vi "VSG25_FM.vi"(0 "Device Handle In":i32, 1 "Run as Subpanel":bool, 2 "FM Cluster In":T1={"Carrier Freq"=1.0, "Baseband Freq"=15.0, "Carrier Hz"=3, "Baseband Hz"=1, "Deviation Freq"=75.0, "Deviation Hz"=1, "Amplitude"=-10.0, "Modulation Shape"=0} {"Modulation Shape" items=["Sine Wave", "Triangle Wave", "Square Wave", "Ramp Wave"]; "Carrier Hz" items=["Hz", "kHz", "MHz", "GHz"]; "Baseband Hz" items=["Hz", "kHz", "MHz", "GHz"]; "Deviation Hz" items=["Hz", "kHz", "MHz", "GHz"]}, 3 "Error In":errorcluster) -> (5 "Device Handle Out":i32, 6 "FM Cluster Out":T1 {"Modulation Shape" items=["Sine Wave", "Triangle Wave", "Square Wave", "Ramp Wave"]; "Carrier Hz" items=["Hz", "kHz", "MHz", "GHz"]; "Baseband Hz" items=["Hz", "kHz", "MHz", "GHz"]; "Deviation Hz" items=["Hz", "kHz", "MHz", "GHz"]}, 7 "Error Out":errorcluster)   [LabVIEW 2014]
uses:
  Frequency Hertz.ctl
  Shape Control.ctl
  FM Cluster.ctl
  sg_lib/VSG25A.lvlib
panel:
  in  "Stop":bool
  out "Device Selected":bool
  in  "Modulation Shape":T3 items=["Sine Wave", "Triangle Wave", "Square Wave", "Ramp Wave"]
  in  "Deviation Hz":T2 items=["Hz", "kHz", "MHz", "GHz"]
  in  "FM Deviation":dbl
  in  "Baseband Hz":T2 items=["Hz", "kHz", "MHz", "GHz"]
  in  "Baseband Frequency":dbl
  in  "RF On":bool
  in  "Carrier Hz":T2 items=["Hz", "kHz", "MHz", "GHz"]
  in  "Amplitude (dBm)":dbl
  in  "Carrier Frequency":dbl
  # "Frequency Modulation"
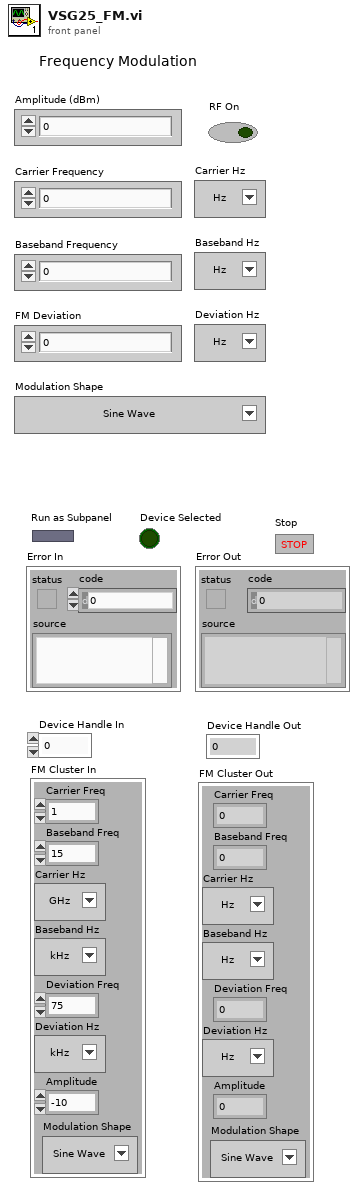
[diagram p1: front panel]
types:
  T1 = typedef "FM Cluster.ctl" = cluster{"Carrier Freq":dbl, "Baseband Freq":dbl, "Carrier Hz":T2, "Baseband Hz":T2, "Deviation Freq":dbl, "Deviation Hz":T2, "Amplitude":dbl, "Modulation Shape":T3}
  T2 = typedef "Frequency Hertz.ctl" = u16
  T3 = typedef "Shape Control.ctl" = u16
  T4 = enum16{"Init", "Proc Events", "Write VSG25", "Exit"}
  T5 = enum32{"Bad", "Idle", "Run top level", "Running"}
  T6 = enum16{"Check Amplitude ", "Check Carrier", "Check Baseband", "Check Deviation", "Stop RF", "Set Freq and Amp", "Set FM", "Finish"}
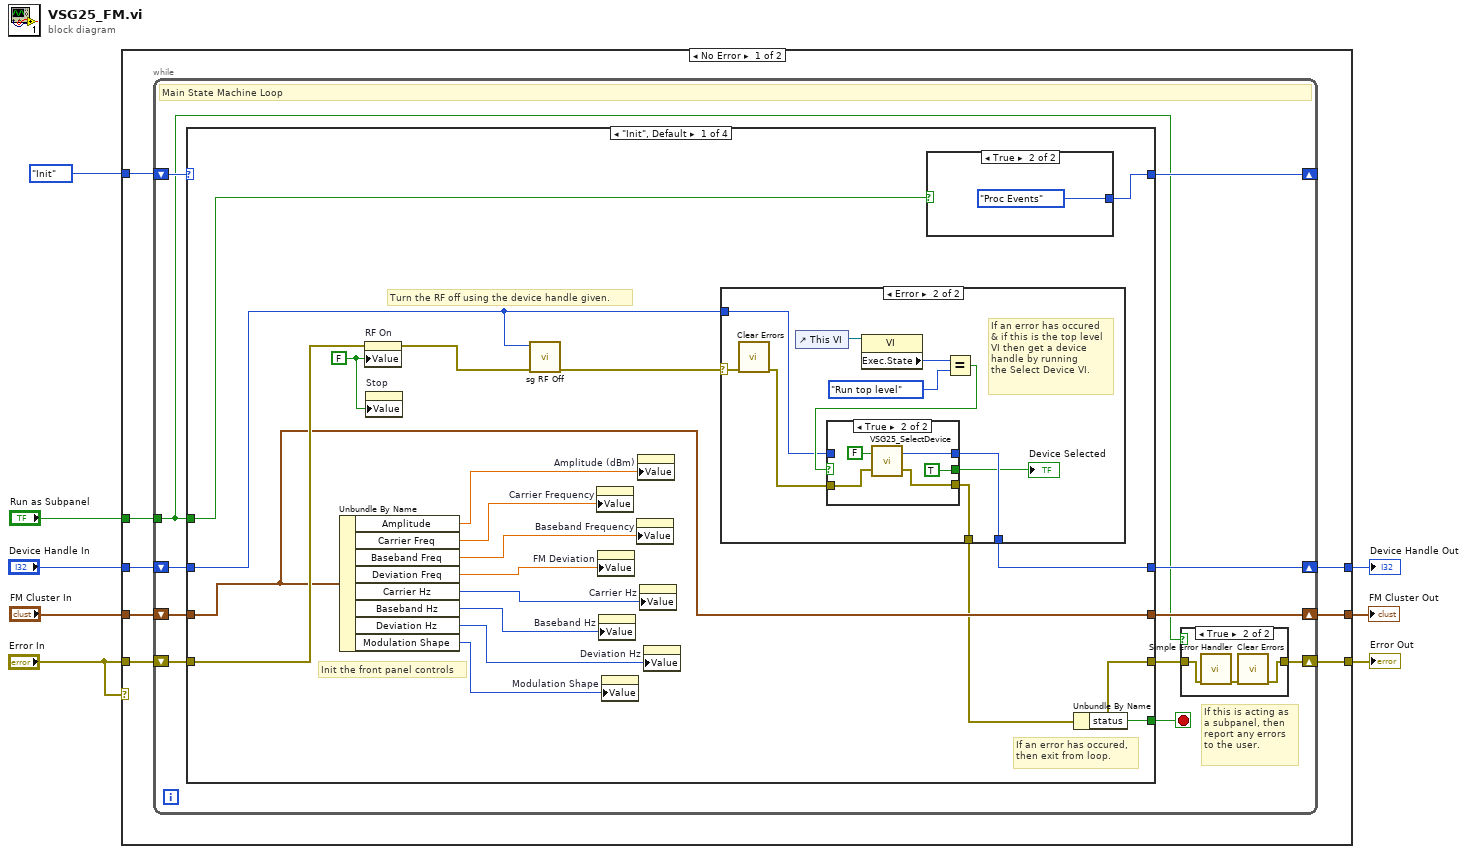
[diagram p0: block diagram]
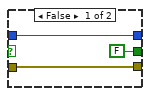
[diagram p4: hidden frame]
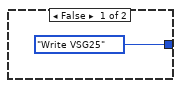
[diagram p5: hidden frame]
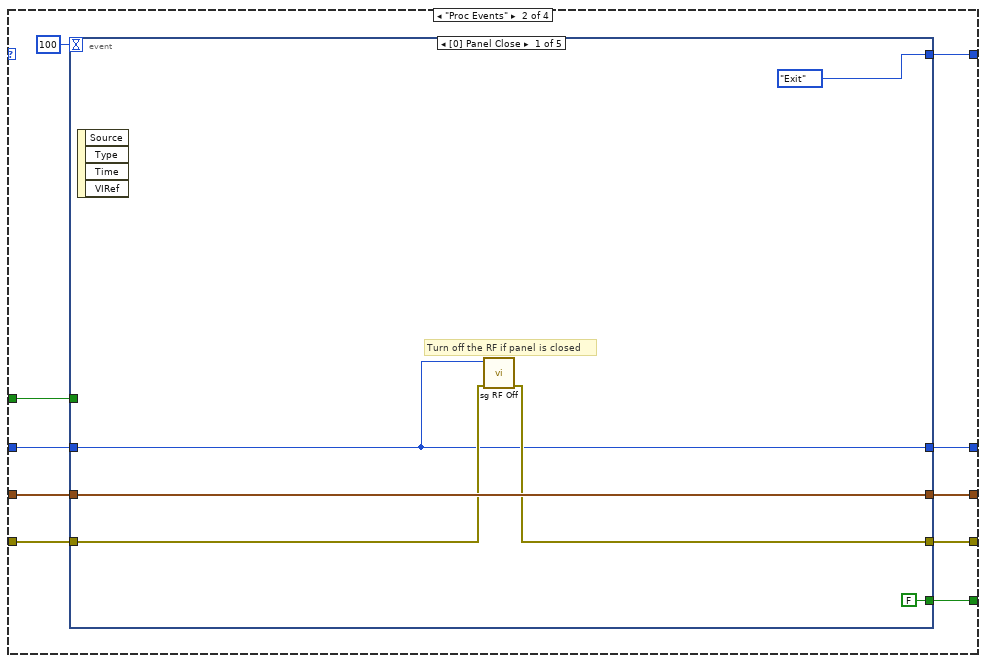
[diagram p6: hidden frame]
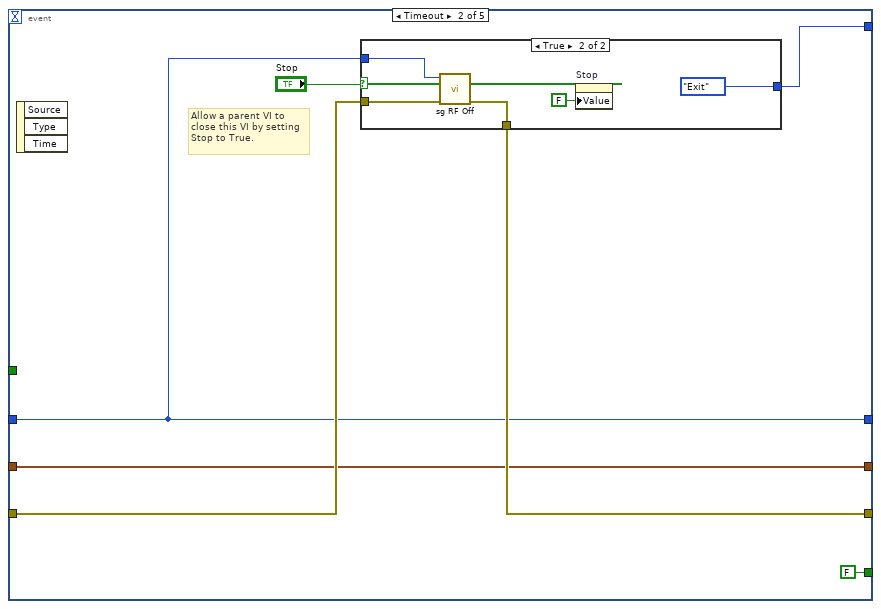
[diagram p7: hidden frame]
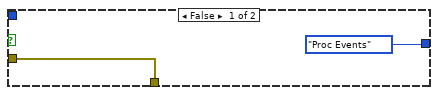
[diagram p8: hidden frame]
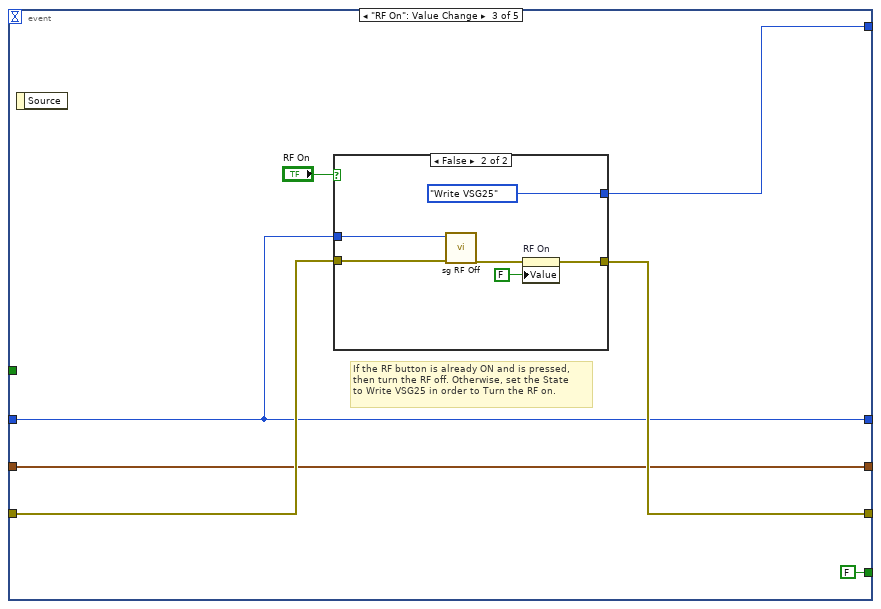
[diagram p9: hidden frame]
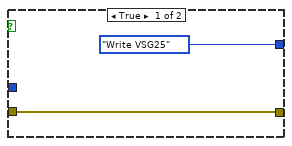
[diagram p10: hidden frame]
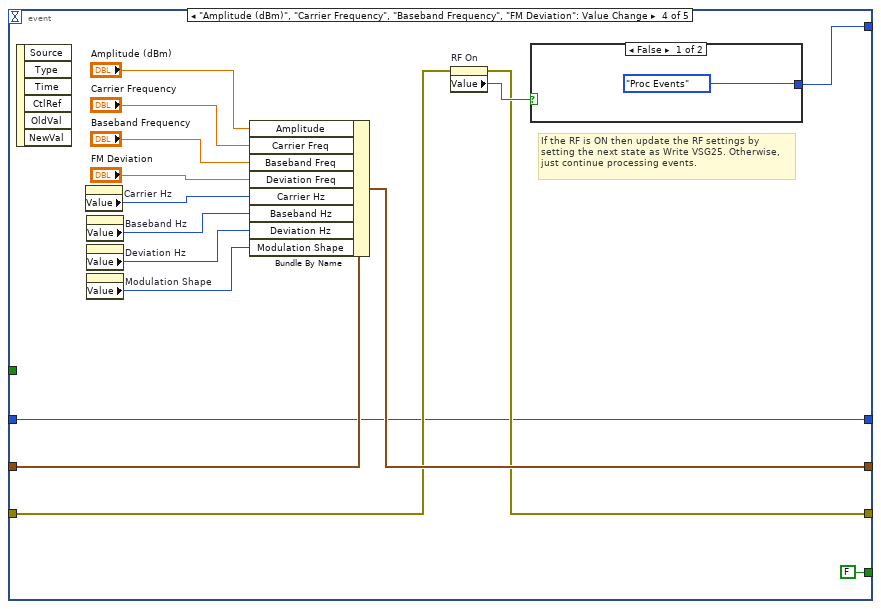
[diagram p11: hidden frame]
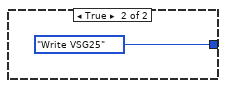
[diagram p12: hidden frame]
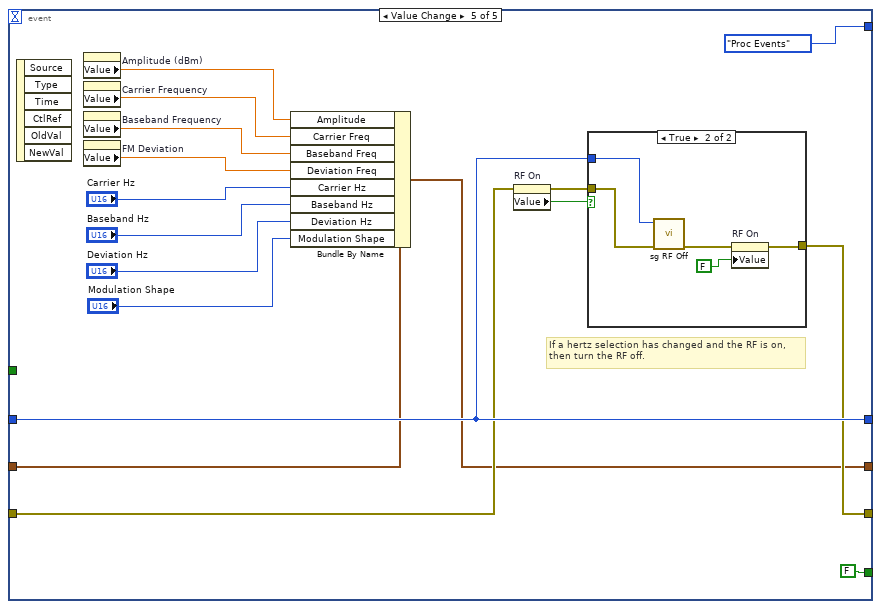
[diagram p13: hidden frame]
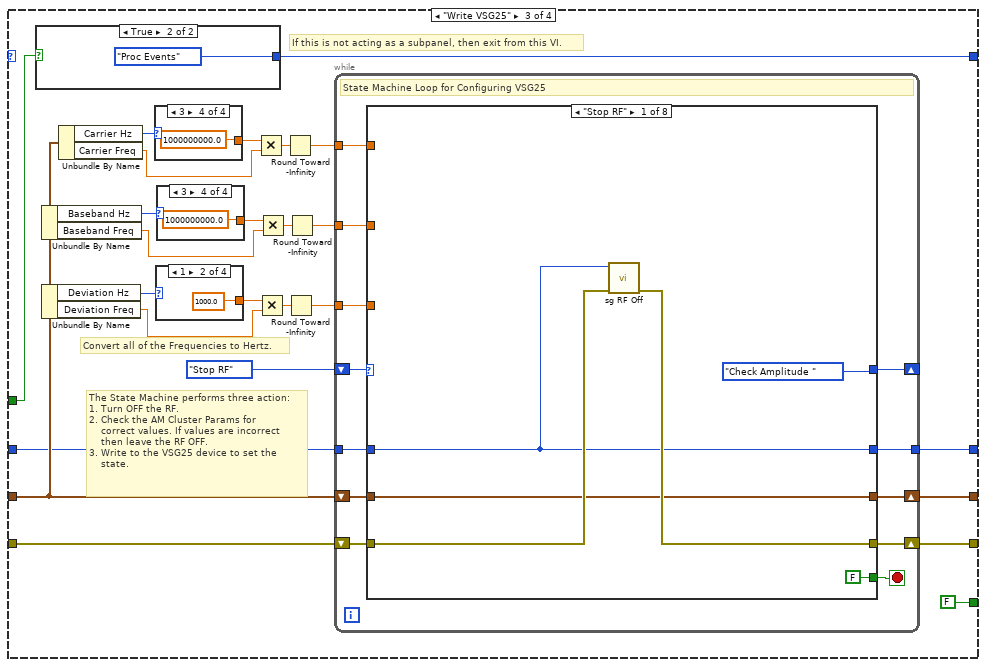
[diagram p15: hidden frame]
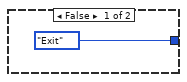
[diagram p16: hidden frame]
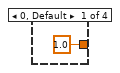
[diagram p17: hidden frame]
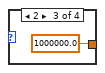
[diagram p18: hidden frame]
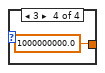
[diagram p19: hidden frame]
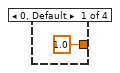
[diagram p20: hidden frame]
diagram:
  n1 = case shown="No Error" "Error In" {
    tunnel: "Error In" -> [w12 w337]
    tunnel: T4."Init" -> [w16 _]
    tunnel: "Run as Subpanel" -> [w15 _]
    tunnel: "Device Handle In" -> [w14 w335]
    tunnel: "FM Cluster In" -> [w13 w336]
    tunnel: [w11 w337] -> w3
    tunnel: [w10 w336] -> w2
    tunnel: [w9 w335] -> w1
    frame No Error {
      n2 = while {
        shift-right: [w26] -> _
        shift-left: w16 -> [w27]
        tunnel: w15 -> [w17]
        shift-right: [w18] -> w11
        shift-left: w12 -> [w23]
        shift-right: [w21] -> w10
        shift-left: w13 -> [w24]
        shift-right: [w20] -> w9
        shift-left: w14 -> [w25]
        stop <- w22 stop-if-true
        # "If this is acting as \na subpanel, then\nreport any errors\nto the user."
        # "Main State Machine Loop"
        n3 = case shown="\"Init\", Default" w27 {
          selector: w27 -> [_ _ _ w330]
          tunnel: [w39 w75 w160 w330] -> w26
          tunnel: w17 -> [w42 w79 w159 _]
          tunnel: w25 -> [w33 w80 w165 w325]
          tunnel: w24 -> [w40 w81 w166 w326]
          tunnel: w23 -> [w41 w82 w170 w327]
          tunnel: [w38 w76 FALSE TRUE] -> w22
          tunnel: [w34 w74 w164 w328] -> w19
          tunnel: [w40 w78 w163 w326] -> w21
          tunnel: [w35 w77 w162 w325] -> w20
          frame "Init", Default {
            w32 = FALSE ("RF On")
            # "Init the front panel controls"
            # "Turn the RF off using the device handle given."
            # "If an error has occured,\nthen exit from loop."
            n4 = Unbundle By Name(w40) -> ("Amplitude"=w50:dbl, "Carrier Freq"=w49:dbl, "Baseband Freq"=w48:dbl, "Deviation Freq"=w47:dbl, "Carrier Hz"=w46:T2, "Baseband Hz"=w45:T2, "Deviation Hz"=w44:T2, "Modulation Shape"=w43:T3)
            n5 = property on="RF On" class="Bool (strict)"(error in=w41, "Value"=w32) -> (error out=w37:errorcluster)  [unwired: 1 in, 1 out]
            n6 = property on="Stop" class="Bool (strict)"("Value"=w32) -> ()  [unwired: 2 in, 2 out]
            n7 = call "sg RF Off.vi"("error in (no error)"=w37, "device"=w33) -> ("error out"=w36:errorcluster)  [unwired: 8 in, 1 out]
            n8 = property on="Carrier Frequency" class="DigNum (strict)"("Value"=w49) -> ()  [unwired: 2 in, 2 out]
            n9 = property on="FM Deviation" class="DigNum (strict)"("Value"=w47) -> ()  [unwired: 2 in, 2 out]
            n10 = property on="Baseband Hz" class="Ring (strict)"("Value"=w45) -> ()  [unwired: 2 in, 2 out]
            n11 = property on="Modulation Shape" class="Ring (strict)"("Value"=w43) -> ()  [unwired: 2 in, 2 out]
            n12 = property on="Baseband Frequency" class="DigNum (strict)"("Value"=w48) -> ()  [unwired: 2 in, 2 out]
            n13 = property on="Amplitude (dBm)" class="DigNum (strict)"("Value"=w50) -> ()  [unwired: 2 in, 2 out]
            n14 = property on="Carrier Hz" class="Ring (strict)"("Value"=w46) -> ()  [unwired: 2 in, 2 out]
            n15 = property on="Deviation Hz" class="Ring (strict)"("Value"=w44) -> ()  [unwired: 2 in, 2 out]
            n16 = case shown="Error" w36 {
              selector: w36 -> [w51 w58]
              tunnel: [w52 w56] -> w35
              tunnel: [w51 w55] -> w34
              tunnel: w33 -> [w52 w54]
              frame No Error {
              }
              frame Error {
                # "If an error has occured\n& if this is the top level\nVI then get a device\nhandle by running \nthe Select Device VI."
                n17 = call <vilib>:"Clear Errors.vi"("error in (no error)"=w58) -> ("error out"=w57:errorcluster)  [unwired: 5 in, 1 out]
                n18 = control-ref of="This VI"() -> (w62:refnum<vi>)
                n19 = property class="VI"(reference=w62) -> ("Exec.State"=w61:T5)  [unwired: 1 in, 2 out]
                n20 = Equal?(x=w61, y=T5."Run top level" ("Execution:State 2")) -> (x = y?=w59:bool)
                n21 = case shown="True" w59 {
                  tunnel: [w65 w70] -> w56
                  tunnel: w54 -> [w65 _]
                  tunnel: w57 -> [w64 w68]
                  tunnel: [w64 w67] -> w55
                  tunnel: [FALSE TRUE] -> w53
                  frame False {
                  }
                  frame True {
                    n22 = call "VSG25_SelectDevice.vi"("ErrorIn"=w68, "AutoSel"=FALSE) -> ("ErrorOut"=w67:errorcluster, "deviceHandle"=w70:i32)
                  }
                }
                "Device Selected" <- w53
              }
            }
            n23 = case shown="True" w42 {
              tunnel: [T4."Write VSG25" T4."Proc Events"] -> w39
              frame False {
              }
              frame True {
              }
            }
            n24 = Unbundle By Name(w34) -> ("status"=w38:bool)
          }
          frame "Proc Events" {
            n25 = event shown="[0] Panel Close" {
              selector: _ -> [_ _ _ _ _]
              dyn-events: _ -> [_ _ _ _ _]
              timeout: 100 -> [_ _ _ _ _]
              tunnel: w82 -> [w85 w92 w108 w121 w148]
              tunnel: w81 -> [w86 w90 w106 w133 w147]
              tunnel: w80 -> [w83 w89 w105 w119 w150]
              tunnel: w79 -> [_ _ _ _ _]
              tunnel: [w84 w91 w107 w120 w149] -> w74
              tunnel: [w86 w90 w106 w132 w146] -> w78
              tunnel: [w83 w89 w105 w119 w150] -> w77
              tunnel: [FALSE FALSE FALSE FALSE FALSE] -> w76
              tunnel: [T4."Exit" w93 w104 w122 T4."Proc Events"] -> w75
              event Panel Close {
                # "Turn off the RF if panel is closed"
                n26 = event-data() -> ()  [unwired: 1 in, 4 out]
                n27 = call "sg RF Off.vi"("error in (no error)"=w85, "device"=w83) -> ("error out"=w84:errorcluster)  [unwired: 8 in, 1 out]
              }
              event Timeout {
                # "Allow a parent VI to \nclose this VI by setting\nStop to True."
                n28 = event-data() -> ()  [unwired: 1 in, 3 out]
                n29 = case shown="True" "Stop" {
                  tunnel: [T4."Proc Events" T4."Exit"] -> w93
                  tunnel: w92 -> [w96 w101]
                  tunnel: [w96 w100] -> w91
                  tunnel: w89 -> [_ w99]
                  frame False {
                  }
                  frame True {
                    n30 = call "sg RF Off.vi"("error in (no error)"=w101, "device"=w99) -> ("error out"=w100:errorcluster)  [unwired: 8 in, 1 out]
                    n31 = property on="Stop" class="Bool (strict)"("Value"=FALSE ("Stop")) -> ()  [unwired: 2 in, 2 out]
                  }
                }
              }
              event "RF On": Value Change {
                # "If the RF button is already ON and is pressed, \nthen turn the RF off. Otherwise, set the State\nto Write VSG25 in order to Turn the RF on."
                n32 = event-data() -> ()  [unwired: 1 in, 1 out]
                n33 = case shown="False" "RF On" {
                  tunnel: [w110 w115] -> w107
                  tunnel: w108 -> [w110 w117]
                  tunnel: w105 -> [_ w116]
                  tunnel: [T4."Write VSG25" T4."Write VSG25"] -> w104
                  frame True {
                  }
                  frame False {
                    n34 = call "sg RF Off.vi"("error in (no error)"=w117, "device"=w116) -> ("error out"=w114:errorcluster)  [unwired: 8 in, 1 out]
                    n35 = property on="RF On" class="Bool (strict)"(error in=w114, "Value"=FALSE ("RF On")) -> (error out=w115:errorcluster)  [unwired: 1 in, 1 out]
                  }
                }
              }
              event "Amplitude (dBm)", "Carrier Frequency", "Baseband Frequency", "FM Deviation": Value Change {
                # "If the RF is ON then update the RF settings by\nsetting the next state as Write VSG25. Otherwise,\njust continue processing events."
                n36 = event-data() -> ()  [unwired: 1 in, 6 out]
                n37 = property on="Carrier Hz" class="Ring (strict)"() -> ("Value"=w127:T2)  [unwired: 2 in, 2 out]
                n38 = property on="Baseband Hz" class="Ring (strict)"() -> ("Value"=w126:T2)  [unwired: 2 in, 2 out]
                n39 = property on="Deviation Hz" class="Ring (strict)"() -> ("Value"=w125:T2)  [unwired: 2 in, 2 out]
                n40 = property on="Modulation Shape" class="Ring (strict)"() -> ("Value"=w124:T3)  [unwired: 2 in, 2 out]
                n41 = Bundle By Name(cluster=w133, "Amplitude"="Amplitude (dBm)", "Carrier Freq"="Carrier Frequency", "Baseband Freq"="Baseband Frequency", "Deviation Freq"="FM Deviation", "Carrier Hz"=w127, "Baseband Hz"=w126, "Deviation Hz"=w125, "Modulation Shape"=w124) -> (w132:T1)
                n42 = property on="RF On" class="Bool (strict)"(error in=w121) -> (error out=w120:errorcluster, "Value"=w123:bool)  [unwired: 1 in, 1 out]
                n43 = case shown="False" w123 {
                  tunnel: [T4."Proc Events" T4."Write VSG25"] -> w122
                  frame False {
                  }
                  frame True {
                  }
                }
              }
              event Value Change {
                # "If a hertz selection has changed and the RF is on,\nthen turn the RF off."
                n44 = event-data() -> ()  [unwired: 1 in, 6 out]
                n45 = property on="Amplitude (dBm)" class="DigNum (strict)"() -> ("Value"=w145:dbl)  [unwired: 2 in, 2 out]
                n46 = property on="Carrier Frequency" class="DigNum (strict)"() -> ("Value"=w144:dbl)  [unwired: 2 in, 2 out]
                n47 = property on="Baseband Frequency" class="DigNum (strict)"() -> ("Value"=w143:dbl)  [unwired: 2 in, 2 out]
                n48 = property on="FM Deviation" class="DigNum (strict)"() -> ("Value"=w142:dbl)  [unwired: 2 in, 2 out]
                n49 = Bundle By Name(cluster=w147, "Amplitude"=w145, "Carrier Freq"=w144, "Baseband Freq"=w143, "Deviation Freq"=w142, "Carrier Hz"="Carrier Hz", "Baseband Hz"="Baseband Hz", "Deviation Hz"="Deviation Hz", "Modulation Shape"="Modulation Shape") -> (w146:T1)
                n50 = property on="RF On" class="Bool (strict)"(error in=w148) -> (error out=w152:errorcluster, "Value"=w151:bool)  [unwired: 1 in, 1 out]
                n51 = case shown="True" w151 {
                  tunnel: [w153 w154] -> w149
                  tunnel: w152 -> [w153 w158]
                  tunnel: w150 -> [_ w157]
                  frame False {
                  }
                  frame True {
                    n52 = call "sg RF Off.vi"("error in (no error)"=w158, "device"=w157) -> ("error out"=w155:errorcluster)  [unwired: 8 in, 1 out]
                    n53 = property on="RF On" class="Bool (strict)"(error in=w155, "Value"=FALSE ("RF On")) -> (error out=w154:errorcluster)  [unwired: 1 in, 1 out]
                  }
                }
              }
            }
          }
          frame "Write VSG25" {
            # "If this is not acting as a subpanel, then exit from this VI."
            # "Convert all of the Frequencies to Hertz."
            # "The State Machine performs three action:\n1. Turn OFF the RF.\n2. Check the AM Cluster Params for \n    correct values. If values are incorrect\n    then leave the RF OFF.\n3. Write to the VSG25 device to set the\n    state."
            n54 = case shown="True" w159 {
              tunnel: [T4."Exit" T4."Proc Events"] -> w160
              frame False {
              }
              frame True {
              }
            }
            n55 = Unbundle By Name(w166) -> ("Baseband Hz"=w176:T2, "Baseband Freq"=w178:dbl)
            n56 = Unbundle By Name(w166) -> ("Deviation Hz"=w172:T2, "Deviation Freq"=w174:dbl)
            n57 = Unbundle By Name(w166) -> ("Carrier Hz"=w182:T2, "Carrier Freq"=w180:dbl)
            n58 = case shown="3" w182 {
              tunnel: [1.0 ("y") 1000.0 ("y") 1000000.0 ("y") 1000000000.0 ("y")] -> w181
              frame 0, Default {
              }
              frame 1 {
              }
              frame 2 {
              }
              frame 3 {
              }
            }
            n59 = case shown="1" w172 {
              tunnel: [1.0 ("y") 1000.0 ("y") 1000000.0 ("y") 1000000000.0 ("y")] -> w173
              frame 0, Default {
              }
              frame 1 {
              }
              frame 2 {
              }
              frame 3 {
              }
            }
            n60 = case shown="3" w176 {
              tunnel: [1.0 ("y") 1000.0 ("y") 1000000.0 ("y") 1000000000.0 ("y")] -> w177
              frame 0, Default {
              }
              frame 1 {
              }
              frame 2 {
              }
              frame 3 {
              }
            }
            n61 = Multiply(x=w181, y=w180) -> (x*y=w183:dbl)
            n62 = Multiply(x=w173, y=w174) -> (x*y=w171:dbl)
            n63 = Multiply(x=w177, y=w178) -> (x*y=w175:dbl)
            n64 = Round Toward -Infinity(1:w183) -> (0:w169:dbl)
            n65 = Round Toward -Infinity(1:w171) -> (0:w167:dbl)
            n66 = Round Toward -Infinity(1:w175) -> (0:w168:dbl)
            n67 = while {
              shift-right: [w194] -> _
              shift-left: T6."Stop RF" -> [w205]
              tunnel: w169 -> [w203]
              tunnel: w168 -> [w202]
              tunnel: w167 -> [w201]
              tunnel: w165 -> [w199]
              tunnel: [w196] -> w162
              shift-right: [w198] -> w164
              shift-left: w170 -> [w204]
              shift-right: [w197] -> w163
              shift-left: w166 -> [w200]
              stop <- w195 stop-if-true
              # "State Machine Loop for Configuring VSG25"
              n68 = case shown="\"Stop RF\"" w205 {
                selector: w205 -> [_ _ _ _ _ _ _ w315]
                tunnel: w204 -> [w211 w213 w242 w260 w278 w300 w309 w312]
                tunnel: w203 -> [_ _ w247 _ _ w298 _ _]
                tunnel: w202 -> [_ _ _ w265 _ _ w311 _]
                tunnel: w201 -> [_ _ _ _ w282 _ w310 _]
                tunnel: w200 -> [w209 w218 w243 w262 w280 w301 w306 w313]
                tunnel: w199 -> [w208 w216 w244 w261 w279 w297 w305 w314]
                tunnel: [w210 w212 w241 w259 w277 w299 w308 w312] -> w198
                tunnel: [w209 w217 w243 w262 w280 w301 w306 w313] -> w197
                tunnel: [w208 w216 w244 w261 w279 w297 w305 w314] -> w196
                tunnel: [FALSE FALSE FALSE FALSE FALSE FALSE FALSE TRUE] -> w195
                tunnel: [T6."Check Amplitude " w214 w248 w264 w283 T6."Set FM" T6."Finish" w315] -> w194
                frame "Stop RF" {
                  n69 = call "sg RF Off.vi"("error in (no error)"=w211, "device"=w208) -> ("error out"=w210:errorcluster)  [unwired: 8 in, 1 out]
                }
                frame "Check Amplitude ", Default {
                  n70 = Unbundle By Name(w218) -> ("Amplitude"=w224:dbl)
                  n71 = Less Or Equal?(x=w224, y=10.0) -> (x <= y?=w220:bool)
                  n72 = Greater Or Equal?(x=w224, y=-80.0) -> (x >= y?=w223:bool)
                  n73 = And(x=w220, y=w223) -> (x .and. y?=w219:bool)
                  n74 = case shown="True" w219 {
                    tunnel: w223 -> [w234 _]
                    tunnel: w224 -> [_ w239]
                    tunnel: w218 -> [w231 w238]
                    tunnel: [w230 w237] -> w217
                    tunnel: [T6."Finish" T6."Check Carrier"] -> w214
                    tunnel: w213 -> [w227 w235]
                    tunnel: [w225 w235] -> w212
                    frame False {
                      n75 = Select(t=10.0, s=w234, f=-80.0) -> (s? t:f=w229:dbl)
                      n76 = Bundle By Name(cluster=w231, "Carrier Freq"=w229) -> (w230:T1)
                      n77 = property on="Amplitude (dBm)" class="DigNum (strict)"("Value"=w229) -> ()  [unwired: 2 in, 2 out]
                      n78 = Merge Errors(w227, errorcluster {"status"=TRUE, "code"=-1, "source"="Invalid Amplitude.\nValue must be between\n-80 dBm and 10 dBm."} ("error constant")) -> (w225:errorcluster)
                    }
                    frame True {
                      n79 = Round Toward -Infinity(1:w239) -> (0:w240:dbl)
                      n80 = Bundle By Name(cluster=w238, "Amplitude"=w240) -> (w237:T1)
                    }
                  }
                }
                frame "Check Carrier" {
                  n81 = Greater Or Equal?(x=w247, y=80000000.0) -> (x >= y?=w252:bool)
                  n82 = Less Or Equal?(x=w247, y=2500000000.0) -> (x <= y?=w246:bool)
                  n83 = Compound Arithmetic op=AND(w252, w246) -> (w251:bool)
                  n84 = case shown="True" w251 {
                    tunnel: [T6."Finish" T6."Check Baseband"] -> w248
                    tunnel: w242 -> [w254 w257]
                    tunnel: [w255 w257] -> w241
                    frame False {
                      n85 = Merge Errors(w254, errorcluster {"status"=TRUE, "code"=-1, "source"="Carrier frequency must \nbe greater than 80 MHz\nand less than 2.5 GHz."} ("error constant")) -> (w255:errorcluster)
                    }
                    frame True {
                    }
                  }
                }
                frame "Check Baseband" {
                  n86 = Greater Or Equal?(x=w265, y=50.0) -> (x >= y?=w270:bool)
                  n87 = Less Or Equal?(x=w265, y=40000000.0) -> (x <= y?=w266:bool)
                  n88 = Compound Arithmetic op=AND(w270, w266) -> (w269:bool)
                  n89 = case shown="False" w269 {
                    tunnel: [T6."Finish" T6."Check Deviation"] -> w264
                    tunnel: w260 -> [w273 w275]
                    tunnel: [w271 w275] -> w259
                    frame False {
                      n90 = Merge Errors(w273, errorcluster {"status"=TRUE, "code"=-1, "source"="Baseband frequency must \nbe greater than 50 Hz\nand less than 40 MHz."} ("error constant")) -> (w271:errorcluster)
                    }
                    frame True {
                    }
                  }
                }
                frame "Check Deviation" {
                  n91 = Greater Or Equal?(x=w282, y=0.0) -> (x >= y?=w288:bool)
                  n92 = Less Or Equal?(x=w282, y=50000000.0) -> (x <= y?=w284:bool)
                  n93 = Compound Arithmetic op=AND(w288, w284) -> (w287:bool)
                  n94 = case shown="True" w287 {
                    tunnel: [T6."Finish" T6."Set Freq and Amp"] -> w283
                    tunnel: w278 -> [w290 w293]
                    tunnel: [w291 w293] -> w277
                    frame False {
                      n95 = Merge Errors(w290, errorcluster {"status"=TRUE, "code"=-1, "source"="Baseband frequency must \nbe greater than 0 Hz\nand less than 50 MHz."} ("error constant")) -> (w291:errorcluster)
                    }
                    frame True {
                    }
                  }
                }
                frame "Set Freq and Amp" {
                  n96 = Unbundle By Name(w301) -> ("Amplitude"=w302:dbl)
                  n97 = call "sg Set Frequency Amplitude.vi"("error in (no error)"=w300, "amplitude"=w302, "frequency"=w298, "device"=w297) -> ("error out"=w299:errorcluster)  [unwired: 6 in, 1 out]
                }
                frame "Set FM" {
                  n98 = Unbundle By Name(w306) -> ("Modulation Shape"=w307:T3)
                  n99 = call "sg Set FM.vi"("shape"=w307, "error in (no error)"=w309, "deviation"=w310, "frequency"=w311, "device"=w305) -> ("error out"=w308:errorcluster)  [unwired: 5 in, 1 out]
                }
                frame "Finish" {
                  # "If no errors have occured, then indicate that the RF is ON."
                  n100 = case shown="Error" w312 {
                    tunnel: [TRUE FALSE] -> w317
                    frame No Error {
                    }
                    frame Error {
                    }
                  }
                  n101 = property on="RF On" class="Bool (strict)"("Value"=w317) -> ()  [unwired: 2 in, 2 out]
                }
              }
            }
          }
          frame "Exit" {
            # "If a device handle was\nacquired using the \nSelect Device VI, then\nclose the handle \nbefore exiting."
            n102 = local read "Device Selected"() -> (w324:bool)
            n103 = case shown="True" w324 {
              tunnel: w325 -> [_ w334]
              tunnel: w327 -> [w331 w333]
              tunnel: [w331 w332] -> w328
              frame False {
              }
              frame True {
                n104 = call "sg Close Device.vi"("error in (no error)"=w333, "device"=w334) -> ("error out"=w332:errorcluster)  [unwired: 8 in, 1 out]
              }
            }
          }
        }
        n105 = case shown="True" w17 {
          tunnel: w19 -> [w28 w30]
          tunnel: [w28 w31] -> w18
          frame False {
          }
          frame True {
            n106 = call <vilib>:"Simple Error Handler.vi"("error in (no error)"=w30) -> ("error out"=w29:errorcluster)  [unwired: 4 in, 4 out]
            n107 = call <vilib>:"Clear Errors.vi"("error in (no error)"=w29) -> ("error out"=w31:errorcluster)  [unwired: 5 in, 1 out]
          }
        }
      }
    }
    frame Error {
    }
  }
  "Error Out" <- w3
  "FM Cluster Out" <- w2
  "Device Handle Out" <- w1
